vi "MaxWait.vi"(0 "WaitLimit (ms)":u32, 2 "StartTick (from outside the node)":u32, 3 "Valeur entrante":bool) -> (1 "break ?":bool)   [LabVIEW 2019]
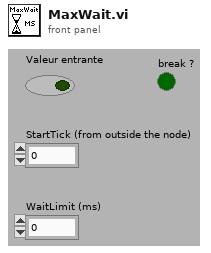
[diagram p1: front panel]
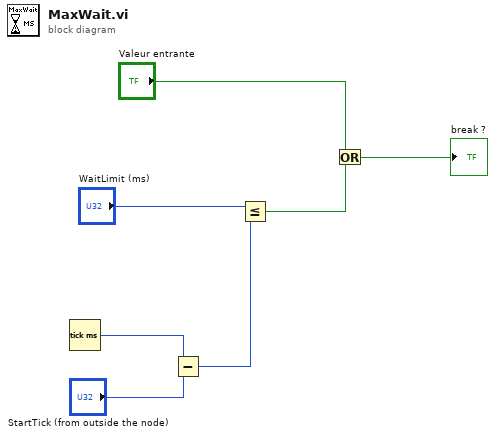
[diagram p0: block diagram]
diagram:
  n1 = Tick Count (ms)() -> (millisecond timer value=w3:u32)
  n2 = Subtract(x=w3, y="StartTick (from outside the node)") -> (x-y=w1:u32)
  n3 = Less Or Equal?(x="WaitLimit (ms)", y=w1) -> (x <= y?=w6:bool)
  n4 = Or(x="Valeur entrante", y=w6) -> (x .or. y?=→"break ?":bool)
